vi "VA显示.vi"(5 "平滑程度":i32=1, 6 "声参数":dbl[](array[numeric])) -> (0 "实时A":dbl, 1 "实时V":dbl, 2 "XY图":cluster{"Value":timestamp[], "Value":dbl[]}[](array[cluster]))   [LabVIEW 2018]
uses:
  gbl.vi
  <vilib>/ptbypt/NI_PtbyPt.lvlib
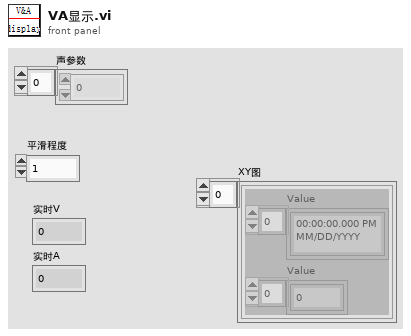
[diagram p1: front panel]
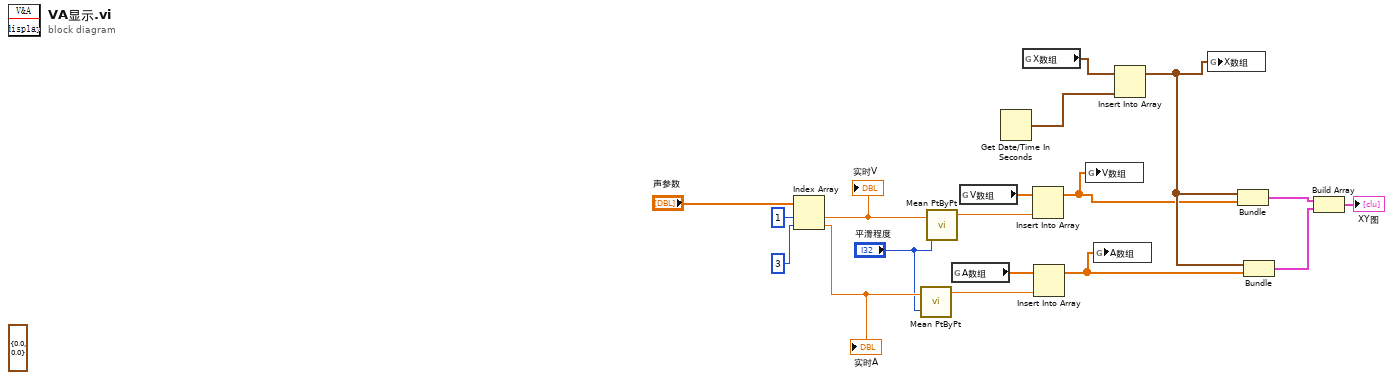
[diagram p0: block diagram]
diagram:
  (unwired) cluster{"V1":dbl, "a":dbl} {"V1"=0.0, "a"=0.0} ("实时监测")
  n1 = Index Array(array="声参数", index #1=1 ("索引"), index #2=3 ("索引")) -> (element #1=w15:dbl, element #2=w14:dbl)
  "实时V" <- w15
  "实时A" <- w14
  n2 = call <vilib>:"Mean PtByPt.vi"("x"=w14, "sample length"="平滑程度") -> ("mean"=w11:dbl)  [unwired: 2 in, 1 out]
  n3 = call <vilib>:"Mean PtByPt.vi"("x"=w15, "sample length"="平滑程度") -> ("mean"=w12:dbl)  [unwired: 2 in, 1 out]
  n4 = global read "gbl.vi" "A数组"() -> (w3:dbl[])
  n5 = global read "gbl.vi" "V数组"() -> (w4:dbl[])
  n6 = Get Date/Time In Seconds() -> (seconds since 1Jan1904=w10:timestamp)
  n7 = global read "gbl.vi" "X数组"() -> (w6:timestamp[])
  n8 = Insert Into Array(array=w4, new element=w12) -> (w2:dbl[])  [unwired: 1 in]
  n9 = Insert Into Array(array=w3, new element=w11) -> (w1:dbl[])  [unwired: 1 in]
  n10 = global write "gbl.vi" "V数组"(w2) -> ()
  n11 = global write "gbl.vi" "A数组"(w1) -> ()
  n12 = Insert Into Array(array=w6, new element=w10) -> (w5:timestamp[])  [unwired: 1 in]
  n13 = global write "gbl.vi" "X数组"(w5) -> ()
  n14 = Bundle("X数组"=w5, "V数组"=w2) -> (w9:cluster{"X数组":timestamp[], "V数组":dbl[]})  [unwired: 1 in]
  n15 = Bundle("X数组"=w5, "A数组"=w1) -> (w8:cluster{"X数组":timestamp[], "A数组":dbl[]})  [unwired: 1 in]
  n16 = Build Array(w9, w8) -> (→"XY图":cluster{"X数组":timestamp[], "A数组":dbl[]}[])
